vi "Data Queue manager.vi"(5 "queue size":i32, 7 "Action":T1=enum."Enqueue", 8 "error in":errorcluster, 11 "Buffer":sgl[](array[numeric])) -> (0 "error out":errorcluster, 1 "# elements in queue":i32, 2 "Empty?":bool, 3 "data out":sgl[](array[numeric]))   [LabVIEW 2018]
uses:
  Controls/Queue Manager Actions.ctl
  Controls/QueueNames.ctl
  Controls/MessagePacket.ctl
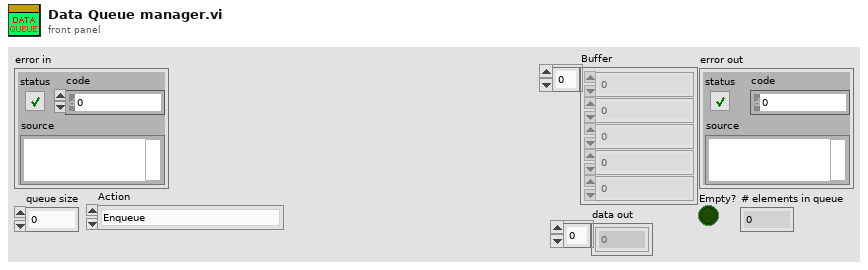
[diagram p1: front panel]
types:
  T1 = typedef "Queue Manager Actions.ctl" = enum16{"Init", "Enqueue", "Enqueue All", "Preview Queue", "Dequeue", "Get Status", "Flush Queue", "Flush All Queues", "Release All Queues", "Release Queue", "Enqueue at Opposite End"}
  T2 = typedef "MessagePacket.ctl" = cluster{"Message":string, "Parameter":variant}
  T3 = typedef "QueueNames.ctl" = enum16{"Main GUI", "Main Scan Processor", "Main Display Processing", "Main Processing", "Main Saving", "Main Display", "Main Table Stage GUI", "Main Table Stage Proc.", "Scan Engine", "Vibratome GUI", "Vibratome Processor", "Slice Engine"}
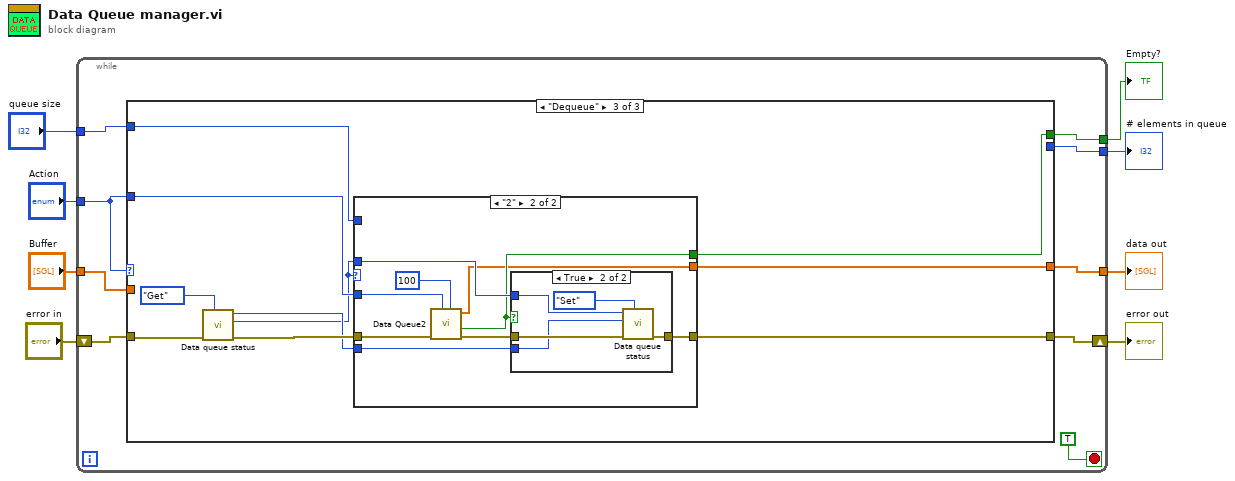
[diagram p0: block diagram]
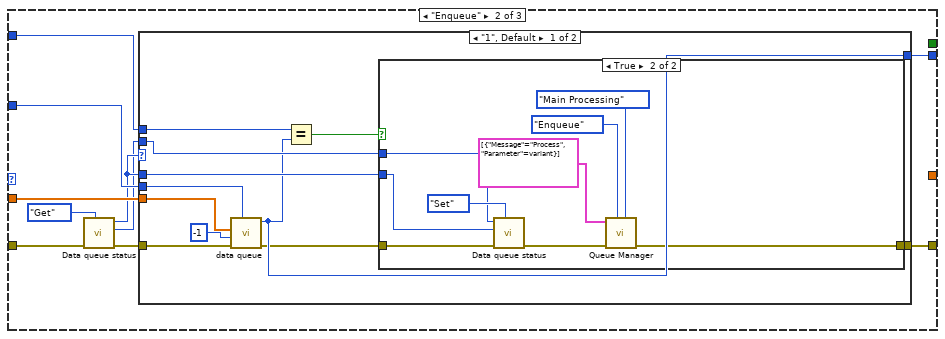
[diagram p3: hidden frame]
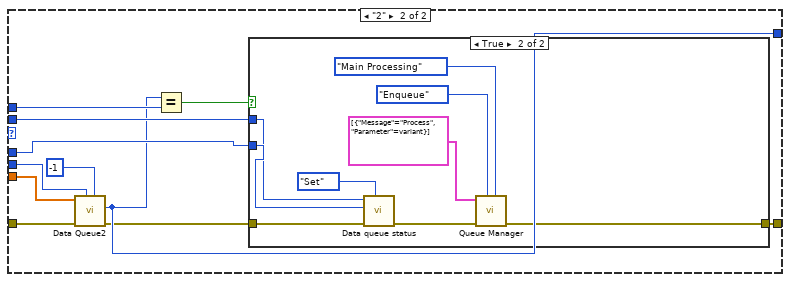
[diagram p5: hidden frame]
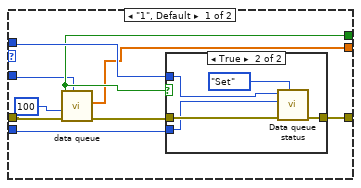
[diagram p7: hidden frame]
diagram:
  n1 = while {
    tunnel: "Buffer" -> [w17]
    tunnel: "Action" -> [w16]
    tunnel: "queue size" -> [w14]
    shift-right: [w13] -> w4
    shift-left: "error in" -> [w15]
    tunnel: [w11] -> w3
    tunnel: [w10] -> w2
    tunnel: [w9] -> w1
    stop <- TRUE stop-if-true
    n2 = case shown="\"Dequeue\"" w16 {
      tunnel: w17 -> [_ w28 _]
      tunnel: w15 -> [w18 w25 w77]
      tunnel: w16 -> [_ w27 w76]
      tunnel: w14 -> [_ w23 w75]
      tunnel: [w18 w20 w74] -> w13
      tunnel: [_ _ w72] -> w11
      tunnel: [_ _ w71] -> w10
      tunnel: [_ w19 _] -> w9
      frame "Init", Default {
      }
      frame "Enqueue" {
        n3 = call "Data queue status.vi"("action"=enum16{"Init", "Get", "Set"}."Get", "error in"=w25) -> ("error out"=w24:errorcluster, "dequeue channel"=w21:enum16{"1", "2"}, "enqueue channel"=w22:enum16{"1", "2"})  [unwired: 7 in]
        n4 = case shown="\"1\", Default" w22 {
          tunnel: w28 -> [w31 w51]
          tunnel: w27 -> [w30 w52]
          tunnel: w24 -> [w38 w60]
          tunnel: w23 -> [w36 w58]
          tunnel: w22 -> [w34 w56]
          tunnel: w21 -> [w35 w55]
          tunnel: [w33 w54] -> w20
          tunnel: [w32 w53] -> w19
          frame "1", Default {
            n5 = call "data queue.vi"("Action"=w30, "error in (no error)"=w38, "timeout in ms (-1)"=-1, "data in"=w31) -> ("error out"=w29:errorcluster, "# elements in queue"=w32:i32)  [unwired: 4 in, 2 out]
            n6 = Equal?(x=w36, y=w32) -> (x = y?=w39:bool)
            n7 = case shown="True" w39 {
              tunnel: [w40 w41] -> w33
              tunnel: w29 -> [w40 w49]
              tunnel: w35 -> [_ w44]
              tunnel: w34 -> [_ w43]
              frame False {
              }
              frame True {
                n8 = call "Data queue status.vi"("action"=enum16{"Init", "Get", "Set"}."Set", "error in"=w49, "dequeue channel"=w43, "enqueue channel"=w44) -> ("error out"=w42:errorcluster)  [unwired: 5 in, 2 out]
                n9 = call "Queue Manager.vi"("Queue Name"=QueueNames."Main Processing", "Action"=Queue_Manager_Actions."Enqueue", "Error In"=w42, "Message Packet Array"=T2[] [{"Message"="Process", "Parameter"=variant}]) -> ("Error Out"=w41:errorcluster)  [unwired: 3 in, 4 out]
              }
            }
          }
          frame "2" {
            n10 = call "Data Queue2.vi"("timeout in ms (-1)"=-1, "Action"=w52, "error in (no error)"=w60, "data in"=w51) -> ("error out"=w50:errorcluster, "# elements in queue"=w53:i32)  [unwired: 4 in, 2 out]
            n11 = Equal?(x=w53, y=w58) -> (x = y?=w57:bool)
            n12 = case shown="True" w57 {
              tunnel: w50 -> [w61 w70]
              tunnel: w56 -> [_ w65]
              tunnel: w55 -> [_ w64]
              tunnel: [w61 w63] -> w54
              frame False {
              }
              frame True {
                n13 = call "Data queue status.vi"("action"=enum16{"Init", "Get", "Set"}."Set", "error in"=w70, "dequeue channel"=w65, "enqueue channel"=w64) -> ("error out"=w62:errorcluster)  [unwired: 5 in, 2 out]
                n14 = call "Queue Manager.vi"("Queue Name"=QueueNames."Main Processing", "Action"=Queue_Manager_Actions."Enqueue", "Error In"=w62, "Message Packet Array"=T2[] [{"Message"="Process", "Parameter"=variant}]) -> ("Error Out"=w63:errorcluster)  [unwired: 3 in, 4 out]
              }
            }
          }
        }
      }
      frame "Dequeue" {
        n15 = call "Data queue status.vi"("action"=enum16{"Init", "Get", "Set"}."Get", "error in"=w77) -> ("error out"=w79:errorcluster, "dequeue channel"=w73:enum16{"1", "2"}, "enqueue channel"=w78:enum16{"1", "2"})  [unwired: 7 in]
        n16 = case shown="\"2\"" w73 {
          tunnel: w76 -> [w82 w103]
          tunnel: w79 -> [w89 w104]
          tunnel: w75 -> [_ _]
          tunnel: w78 -> [w86 w100]
          tunnel: w73 -> [w87 w99]
          tunnel: [w85 w98] -> w74
          tunnel: [w84 w97] -> w72
          tunnel: [w83 w96] -> w71
          frame "1", Default {
            n17 = call "data queue.vi"("Action"=w82, "error in (no error)"=w89, "timeout in ms (-1)"=100) -> ("error out"=w81:errorcluster, "data out"=w83:sgl[], "Empty?"=w84:bool)  [unwired: 5 in, 1 out]
            n18 = case shown="True" w84 {
              tunnel: [w90 w94] -> w85
              tunnel: w81 -> [w90 w93]
              tunnel: w87 -> [_ w92]
              tunnel: w86 -> [_ w91]
              frame False {
              }
              frame True {
                n19 = call "Data queue status.vi"("action"=enum16{"Init", "Get", "Set"}."Set", "error in"=w93, "dequeue channel"=w91, "enqueue channel"=w92) -> ("error out"=w94:errorcluster)  [unwired: 5 in, 2 out]
              }
            }
          }
          frame "2" {
            n20 = call "Data Queue2.vi"("timeout in ms (-1)"=100, "Action"=w103, "error in (no error)"=w104) -> ("error out"=w101:errorcluster, "Empty?"=w97:bool, "data out"=w96:sgl[])  [unwired: 5 in, 1 out]
            n21 = case shown="True" w97 {
              tunnel: w101 -> [w105 w109]
              tunnel: w100 -> [_ w108]
              tunnel: w99 -> [_ w107]
              tunnel: [w105 w106] -> w98
              frame False {
              }
              frame True {
                n22 = call "Data queue status.vi"("action"=enum16{"Init", "Get", "Set"}."Set", "error in"=w109, "dequeue channel"=w108, "enqueue channel"=w107) -> ("error out"=w106:errorcluster)  [unwired: 5 in, 2 out]
              }
            }
          }
        }
      }
    }
  }
  "error out" <- w4
  "Empty?" <- w3
  "data out" <- w2
  "# elements in queue" <- w1
